vi "Calibration.vi"() -> ()   [LabVIEW 2016]
uses:
  controls/EnumFGVHDT.ctl
  controls/Enum.ctl
  Course Project/support/Message Queue/Message Cluster.ctl
  <vilib>/rvi/errors/niLvFpgaAdjustHostInterfaceError.vi
  <vilib>/Utility/config.llb/Read Key (Double).vi
  <vilib>/Utility/config.llb/Read Key (String).vi
  <vilib>/Utility/config.llb/Read Key (U32).vi
  <vilib>/Utility/config.llb/Write Key (Double).vi
  <vilib>/Utility/config.llb/Write Key (String).vi
  <vilib>/Utility/config.llb/Write Key (Boolean).vi
  controls/FPGAVIreferenceTypeDef.ctl
  <vilib>/rvi/interface/nirviReadWriteControl/nirviReadWriteControl.xnode
  FPGA Bitfiles/qnmController797_usbRio80MHz_1.lvbitx
  <vilib>/regexp/Match Regular Expression.xnode
  Course Project/support/Message Queue/Message Queue.lvlib
  Course Project/support/User Event - Stop/User Event - Stop.lvlib
  <vilib>/Utility/config.llb/NI_LVConfig.lvlib
  NiFpgaLv.dll
panel:
  in  "Actions":i32(listbox)
  in  "Menus":T1(tab)
  in  "ActionsCalib":T2={"Calibrations"=0, "Calib parameters"={"Sensitivity"={"Sens X"=1e-07, "Sens Y"=1e-07, "Sens Z"=2e-08}, "Range"={"Range X"=0.0, "Range Y"=0.0, "Range Z"=0.0}, "Gain"={"HV gain X"=0.0, "HV gain Y"=0.0, "HV gain Z"=0.0}}, "EditList"={"Add"=FALSE, "Copy"=FALSE, "Delete"=FALSE, "Up"=FALSE, "Down"=FALSE, "Apply"=FALSE}} {"Calib parameters"."Gain"."HV gain X" min=0.0 max=44.0 step=1.0 format="%#.0f"; "Calib parameters"."Gain"."HV gain Y" min=0.0 max=44.0 step=1.0 format="%#.0f"; "Calib parameters"."Gain"."HV gain Z" min=0.0 max=44.0 step=1.0 format="%#.0f"; "Calib parameters"."Range"."Range X" format="%#_3pm"; "Calib parameters"."Range"."Range Y" format="%#_3pm"; "Calib parameters"."Range"."Range Z" format="%#_3pm"; "Calib parameters"."Sensitivity"."Sens X" format="%#.2pm/V"; "Calib parameters"."Sensitivity"."Sens Y" format="%#.2pm/V"; "Calib parameters"."Sensitivity"."Sens Z" format="%#.2pm/V"}
  in  "OpenHysteresisVi":bool
  out "fwd":dbl[](array[numeric]) format="%#.4g"
  out "bwd":dbl[](array[numeric]) format="%#.4g"
  in  "Hyst Compens":cluster{"Hysteresis Comp":bool}={"Hysteresis Comp"=TRUE}
  in  "Voltage Limits":cluster{"X":dbl, "Y":dbl, "Z":dbl}={"X"=10.0, "Y"=10.0, "Z"=10.0} {"Z" min=-10.0 max=10.0 format="%#_3pV"; "Y" min=-10.0 max=10.0 format="%#_3pV"; "X" min=-10.0 max=10.0 format="%#_3pV"}
  in  "HV":T3
  in  "Analogs":T4={"AI"={"0"=TRUE, "1"=TRUE, "2"=TRUE, "3"=TRUE, "4"=TRUE, "5"=TRUE, "6"=TRUE}, "AO"={"0"=TRUE, "1"=TRUE, "2"=TRUE, "3"=TRUE, "4"=TRUE, "5"=TRUE, "6"=TRUE}}
  in  "ScannerConfig":T5={"Speed config"=FALSE, "Time Constant (us)"=40} {"Time Constant (us)" format="%#.0f"}
  # "Piezo Calibration"
  # "Polynom coeff : a+bx +cx2+dx3"
  # "Hysteresis Compensation"
  # "High Voltage"
  # "between -10V..+10V"
  # "AI/AO inversion"
  # "Non inverted"
  # "Inverted"
  # "Non inverted"
  # "Inverted"
  # "Scanner Configuration"
  # "- slow"
  # "- fast"
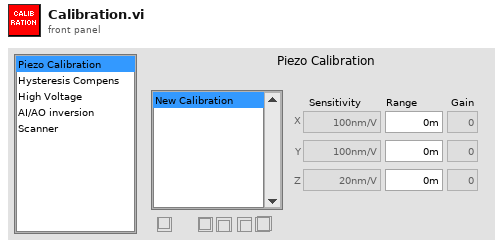
[diagram p1: front panel]
types:
  T1 = enum32{"Piezo Calibration", "Hyst Compens", "High Voltage", "Hyst Compens 2", "Hyst Compens 3", "High Voltage 2", "High Voltage 3", "High Voltage 4", "High Voltage 5"}
  T2 = cluster{"Calibrations":i32, "Calib parameters":cluster{"Sensitivity":cluster{"Sens X":dbl, "Sens Y":dbl, "Sens Z":dbl}, "Range":cluster{"Range X":dbl, "Range Y":dbl, "Range Z":dbl}, "Gain":cluster{"HV gain X":dbl, "HV gain Y":dbl, "HV gain Z":dbl}}, "EditList":cluster{"Add":bool, "Copy":bool, "Delete":bool, "Up":bool, "Down":bool, "Apply":bool}}
  T3 = cluster{"X":bool, "Y":bool, "Z":bool, "X 2":bool, "Y 2":bool, "Z 2":bool}
  T4 = cluster{"AI":cluster{"0":bool, "1":bool, "2":bool, "3":bool, "4":bool, "5":bool, "6":bool}, "AO":cluster{"0":bool, "1":bool, "2":bool, "3":bool, "4":bool, "5":bool, "6":bool}}
  T5 = cluster{"Speed config":bool, "Time Constant (us)":u16}
  T6 = typedef "EnumFGVHDT.ctl" = enum16{"Init", "Read", "Write", "Push", "Pop"}
  T7 = typedef "Message Queue.lvlib/All Message Queues.ctl" = cluster{"IU":refnum<queue>}
  T8 = typedef "Enum.ctl" = enum16{"Init", "Read", "Write"}
  T9 = enum16{"fractional", "engineering", "exponential"}
  T10 = typedef "Message Queue.lvlib/Message Cluster.ctl" = cluster{"Message":string, "Données de message":variant}
  T11 = cluster{"Sensitivity":cluster{"Sens Z":dbl, "Sens Y":dbl, "Sens X":dbl}, "Range":cluster{"Range Z":dbl, "Range Y":dbl, "Range X":dbl}, "HV gain":cluster{"HV gain Z":i32, "HV gain Y":i32, "HV gain X":i32}}
  T12 = cluster{"calibName":string[], "calibParameters":cluster{"Sensitivity":cluster{"Sens X":dbl, "Sens Y":dbl, "Sens Z":dbl}, "Range":cluster{"Range X":dbl, "Range Y":dbl, "Range Z":dbl}, "HV gain":cluster{"HV gain X":dbl, "HV gain Y":dbl, "HV gain Z":dbl}}[], "calibIndex":i32}
  T13 = typedef "NI_LVConfig.lvlib/Config Data RefNum.ctl" = refnum<k1>
  T14 = cluster{"Sensitivity":cluster{"Sens X":dbl, "Sens Y":dbl, "Sens Z":dbl}, "Range":cluster{"Range X":dbl, "Range Y":dbl, "Range Z":dbl}, "HV gain":cluster{"HV gain X":dbl, "HV gain Y":dbl, "HV gain Z":dbl}}[]
  T15 = cluster{"Sensitivity":cluster{"Sens X":dbl, "Sens Y":dbl, "Sens Z":dbl}, "Range":cluster{"Range X":dbl, "Range Y":dbl, "Range Z":dbl}, "HV gain":cluster{"HV gain X":dbl, "HV gain Y":dbl, "HV gain Z":dbl}}
  T16 = cluster{"Sens X":dbl, "Sens Y":dbl, "Sens Z":dbl}
  T17 = cluster{"Range X":dbl, "Range Y":dbl, "Range Z":dbl}
  T18 = cluster{"HV gain X":dbl, "HV gain Y":dbl, "HV gain Z":dbl}
  T19 = cluster{"Sensitivity":cluster{"Sens X":dbl, "Sens Y":dbl, "Sens Z":dbl}, "Range":cluster{"Range X":dbl, "Range Y":dbl, "Range Z":dbl}, "Gain":cluster{"HV gain X":dbl, "HV gain Y":dbl, "HV gain Z":dbl}}
  T20 = typedef "FPGAVIreferenceTypeDef.ctl" = refnum<k20>
  T21 = cluster{"0":bool, "1":bool, "2":bool, "3":bool, "4":bool, "5":bool, "6":bool}
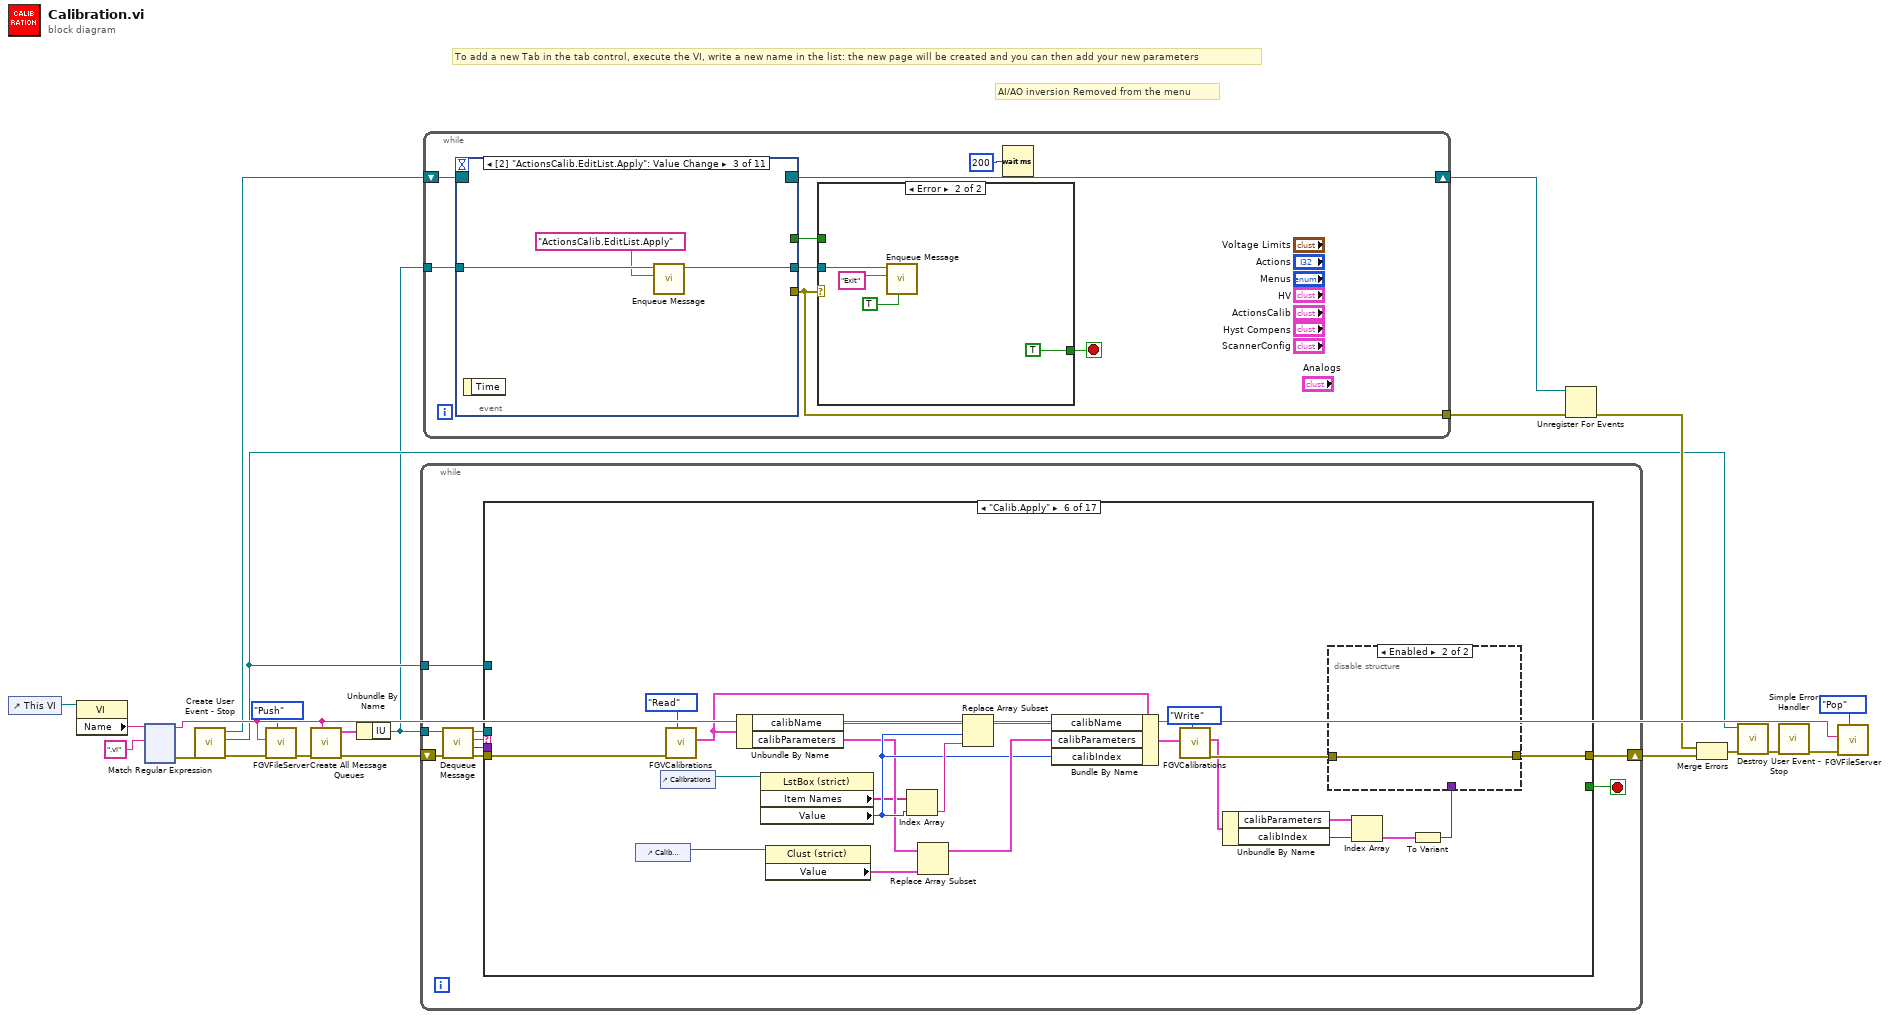
[diagram p0: block diagram]
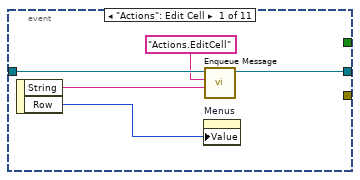
[diagram p3: hidden frame]
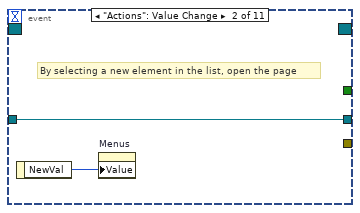
[diagram p4: hidden frame]
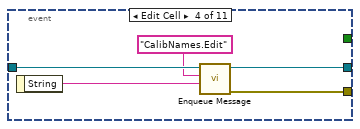
[diagram p5: hidden frame]
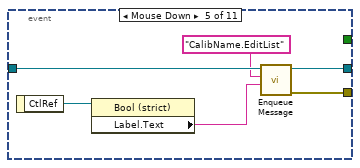
[diagram p6: hidden frame]
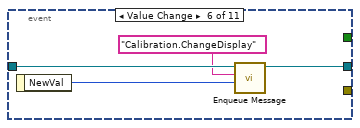
[diagram p7: hidden frame]
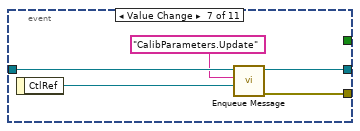
[diagram p8: hidden frame]
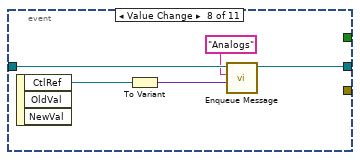
[diagram p9: hidden frame]
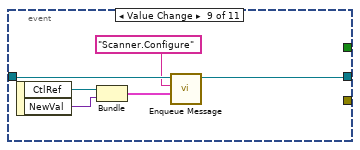
[diagram p10: hidden frame]
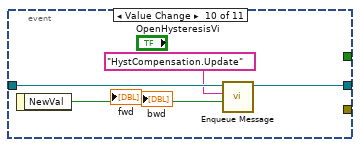
[diagram p11: hidden frame]
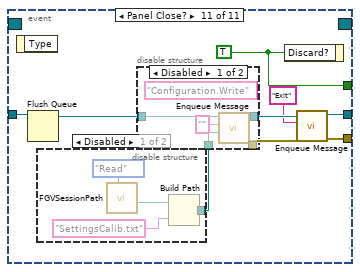
[diagram p12: hidden frame]
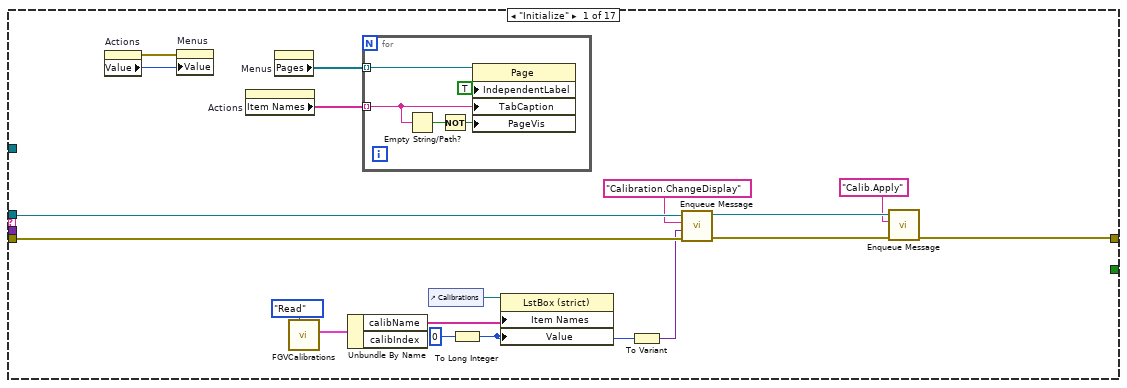
[diagram p15: hidden frame]
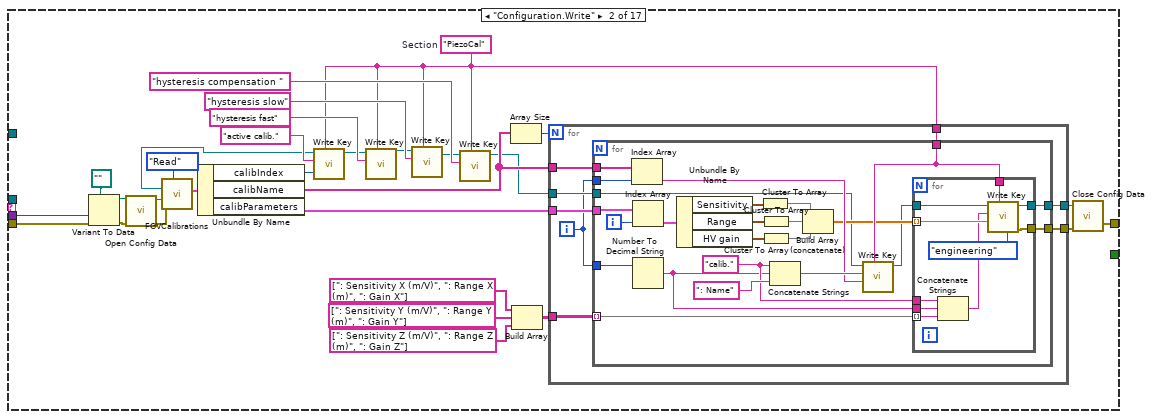
[diagram p16: hidden frame]
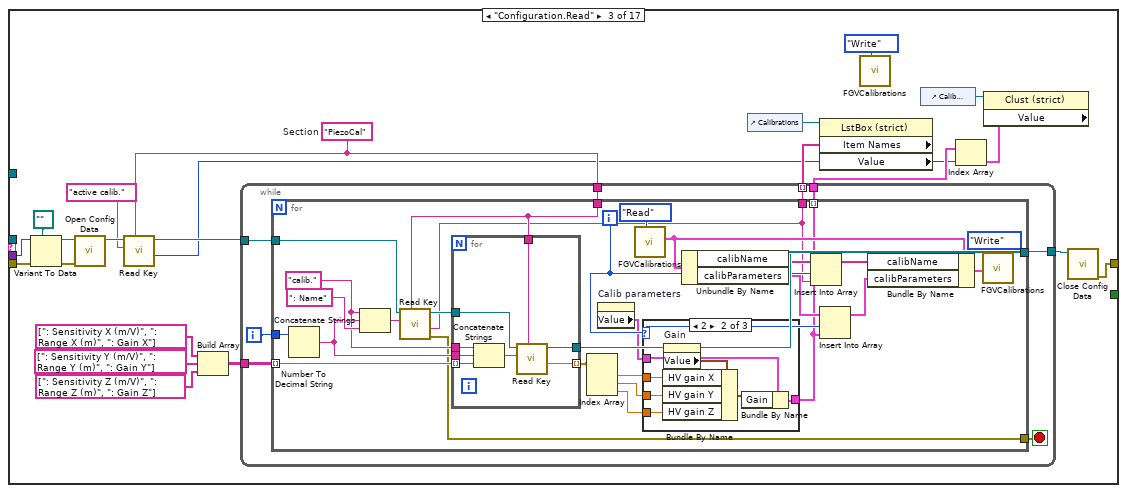
[diagram p17: hidden frame]
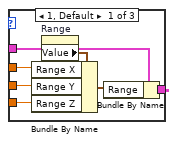
[diagram p18: hidden frame]
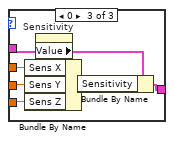
[diagram p19: hidden frame]
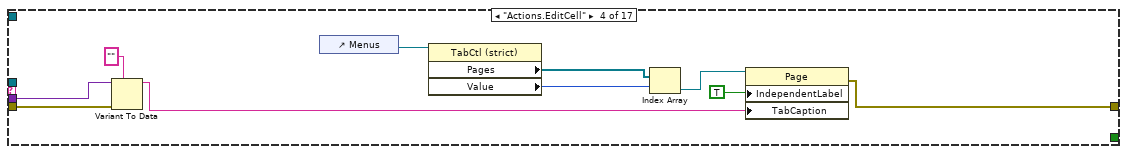
[diagram p20: hidden frame]
diagram:
  # "AI/AO inversion Removed from the menu"
  # "To add a new Tab in the tab control, execute the VI, write a new name in the list: the new page will be created and you can then add your new parameters"
  n1 = control-ref of="This VI"() -> (w9:refnum<vi>)
  n2 = property class="VI"(reference=w9) -> ("Name"=w8:string)  [unwired: 1 in, 2 out]
  n3 = xnode "Match Regular Expression"("input string"=w8, "regular expression"=".vi") -> ("before match"=w21:string, "error out"=w6:errorcluster)  [unwired: 4 in, 3 out]
  n4 = call "Create User Event - Stop.vi"("entrée d'erreur (pas d'erreur)"=w6) -> ("sortie d'erreur"=w4:errorcluster, "Événement utilisateur - Arrêt"=w17:refnum<user-event>, "Refnum Enregistrement à l'événement Arrêt"=w14:refnum<event-registration>)  [unwired: 8 in]
  n5 = call "FGVFileServer.vi"("Enum"=EnumFGVHDT."Push", "error in"=w4, "New VI"=w21) -> ("error out"=w3:errorcluster)  [unwired: 7 in, 1 out]
  n6 = call "Create All Message Queues.vi"("QueueName"=w21, "ErrorIn"=w3) -> ("ErrorOut"=w10:errorcluster, "MessageQueueOut"=w11:T7)  [unwired: 8 in]
  n7 = Unbundle By Name(w11) -> ("IU"=w13:refnum<queue>)
  n8 = while {
    tunnel: w13 -> [w22]
    tunnel: w17 -> [w28]
    shift-right: [w29] -> w12
    shift-left: w10 -> [w27]
    stop <- w30 stop-if-true
    n9 = call "Dequeue Message.vi"("entrée d'erreur (pas d'erreur)"=w27, "File d'attente de messages"=w22) -> ("sortie d'erreur"=w26:errorcluster, "Données de message"=w24:variant, "Message"=w25:string, "File d'attente de message dup."=w23:refnum<queue>)  [unwired: 6 in]
    n10 = case "Conditions des messages" shown="\"Calib.Apply\"" w25 {
      selector: w25 -> [_ _ _ _ _ _ _ _ _ _ _ _ _ _ _ _ w601]
      tunnel: w23 -> [w47 _ _ _ w242 _ _ _ _ w403 _ _ _ w558 _ w597 _]
      tunnel: w26 -> [w41 w62 w148 w222 w233 w258 w296 w302 w393 w398 w414 w517 w525 w557 w590 w593 _]
      tunnel: [w38 w59 w128 w217 w235 w256 w290 w298 w386 w399 w411 w517 w519 w542 w585 w594 w599] -> w29
      tunnel: [_ _ _ _ _ _ _ _ _ _ _ _ _ _ _ TRUE _] -> w30
      tunnel: w24 -> [_ w55 w147 w221 _ _ w295 w301 w392 w395 w413 _ w526 w556 w589 _ _]
      tunnel: w28 -> [_ _ _ _ _ _ _ _ _ _ _ _ _ _ _ w592 _]
      frame "Initialize" {
        n11 = property on="Actions" class="LstBox (strict)"() -> (error out=w43:errorcluster, "Value"=w44:i32)  [unwired: 2 in, 1 out]
        n12 = property on="Menus" class="TabCtl (strict)"(error in=w43, "Value"=w44) -> ()  [unwired: 1 in, 2 out]
        n13 = property on="Actions" class="LstBox (strict)"() -> ("Item Names"=w46:string[])  [unwired: 2 in, 2 out]
        n14 = property on="Menus" class="TabCtl (strict)"() -> ("Pages"=w45:refnum<vi>[])  [unwired: 2 in, 2 out]
        n15 = call "FGVCalibrations.vi"("Enum"=Enum."Read") -> ("calibOut"=w34:T12)  [unwired: 9 in, 1 out]
        n16 = Unbundle By Name(w34) -> ("calibName"=w32:string[])  [unwired: 1 out]
        n17 = for {
          tunnel: w45 -> [w53] mode=indexing
          tunnel: w46 -> [w49] mode=indexing
          n18 = Empty String/Path?(string/path=w49) -> (empty?=w51:bool)
          n19 = Not(x=w51) -> (.not. x?=w50:bool)
          n20 = property class="Page"(reference=w53, "IndependentLabel"=TRUE ("Étiquette indépendante"), "TabCaption"=w49, "PageVis"=w50) -> ()  [unwired: 1 in, 2 out]
        }
        n21 = control-ref of="Calibrations"() -> (w33:refnum<vi>)
        n22 = To Long Integer(number=0) -> (32bit integer=w40:i32)
        n23 = property class="LstBox (strict)"(reference=w33, "Item Names"=w32, "Value"=w40) -> ()  [unwired: 1 in, 2 out]
        n24 = To Variant(anything=w40) -> (Variant=w36:variant)
        n25 = call "Enqueue Message.vi"("error in"=w41, "Data"=w36, "Message"="Calibration.ChangeDisplay", "Queue"=w47) -> ("error out"=w39:errorcluster, "Queue dup."=w48:refnum<queue>)  [unwired: 6 in]
        n26 = call "Enqueue Message.vi"("error in"=w39, "Message"="Calib.Apply", "Queue"=w48) -> ("error out"=w38:errorcluster)  [unwired: 7 in, 1 out]
      }
      frame "Configuration.Write" {
        w66 = "PiezoCal"  # Section
        n27 = Variant To Data(error in=w62, type=path "" ("appended path"), Variant=w55) -> (data=w56:path, error out=w61:errorcluster)
        n28 = call <vilib>:"Open Config Data.vi"("error in (no error)"=w61, "configuration file path"=w56) -> ("error out"=w58:errorcluster, "refnum"=w57:T13)  [unwired: 1 in, 7 out]
        n29 = call "FGVCalibrations.vi"("Enum"=Enum."Read", "error in"=w58) -> ("calibOut"=w74:T12)  [unwired: 8 in, 1 out]
        n30 = Unbundle By Name(w74) -> ("calibIndex"=w64:i32, "calibName"=w78:string[], "calibParameters"=w65:T14)
        n31 = call-poly <vilib>:"Write Key.vi"("section"=w66, "value"=w64, "key"="active calib.", "refnum"=w57) -> ("refnum out"=w67:T13)  [unwired: 4 in, 3 out]
        n32 = call-poly <vilib>:"Write Key.vi"("section"=w66, "key"="hysteresis fast", "refnum"=w67) -> ("refnum out"=w68:T13)  [unwired: 2 in, 6 out]
        n33 = call-poly <vilib>:"Write Key.vi"("section"=w66, "key"="hysteresis slow", "refnum"=w68) -> ("refnum out"=w69:T13)  [unwired: 2 in, 6 out]
        n34 = call-poly <vilib>:"Write Key.vi"("section"=w66, "key"="hysteresis compensation ", "refnum"=w69) -> ("refnum out"=w76:T13)  [unwired: 2 in, 6 out]
        n35 = Array Size(array=w78) -> (size(s)=w77:i32)
        n36 = Build Array(string[] [": Sensitivity X (m/V)", ": Range X (m)", ": Gain X"] ("Array"), string[] [": Sensitivity Y (m/V)", ": Range Y (m)", ": Gain Y"] ("Array"), string[] [": Sensitivity Z (m/V)", ": Range Z (m)", ": Gain Z"] ("Array")) -> (w79:string[][])
        n37 = for {
          N: w77 -> [_]
          tunnel: w65 -> [w90]
          tunnel: w79 -> [w89]
          tunnel: w66 -> [w88]
          tunnel: w78 -> [w86]
          tunnel: w76 -> [w87]
          tunnel: [w84] -> w60
          tunnel: [w83] -> w54
          i -> [w85]
          n38 = for {
            tunnel: w86 -> [w114]
            tunnel: w90 -> [w110]
            tunnel: w88 -> [w108]
            tunnel: w89 -> [w93] mode=indexing
            tunnel: w87 -> [w100]
            tunnel: w85 -> [w98]
            tunnel: w85 -> [w97]
            tunnel: [w92] -> w84
            tunnel: [w91] -> w83
            i -> [w96]
            w95 = "calib."
            n39 = Index Array(array=w114, index=w97) -> (element=w111:string)
            n40 = Index Array(array=w110, index=w96) -> (element=w109:T15)
            n41 = Number To Decimal String(number=w98) -> (decimal integer string=w94:string)  [unwired: 1 in]
            n42 = Unbundle By Name(w109) -> ("Sensitivity"=w107:T16, "Range"=w105:T17, "HV gain"=w106:T18)
            n43 = Cluster To Array(cluster=w107) -> (array=w104:dbl[])
            n44 = Cluster To Array(cluster=w105) -> (array=w103:dbl[])
            n45 = Cluster To Array(cluster=w106) -> (array=w102:dbl[])
            n46 = Concatenate Strings(w95, w94, ": Name") -> (w112:string)
            n47 = Build Array (concatenate)(w104, w103, w102) -> (w101:dbl[])
            n48 = call-poly <vilib>:"Write Key.vi"("section"=w108, "value"=w111, "key"=w112, "refnum"=w100) -> ("refnum out"=w99:T13)  [unwired: 2 in, 5 out]
            n49 = for {
              tunnel: w108 -> [w124]
              tunnel: w101 -> [w123] mode=indexing
              tunnel: w99 -> [w122]
              tunnel: w95 -> [w121]
              tunnel: w94 -> [w120]
              tunnel: w93 -> [w119] mode=indexing
              tunnel: [w117] -> w92
              tunnel: [w116] -> w91
              n50 = Concatenate Strings(w121, w120, w119) -> (w118:string)
              n51 = call-poly <vilib>:"Write Key.vi"("format (fractional)"=T9."engineering", "section"=w124, "value"=w123, "key"=w118, "refnum"=w122) -> ("error out"=w117:errorcluster, "refnum out"=w116:T13)  [unwired: 3 in, 2 out]
            }
          }
        }
        n52 = call <vilib>:"Close Config Data.vi"("error in (no error)"=w60, "refnum"=w54) -> ("error out"=w59:errorcluster)  [unwired: 1 in, 8 out]
      }
      frame "Configuration.Read" {
        w141 = "PiezoCal"  # Section
        n53 = Variant To Data(error in=w148, type=path "" ("appended path"), Variant=w147) -> (data=w149:path, error out=w150:errorcluster)
        n54 = call <vilib>:"Open Config Data.vi"("error in (no error)"=w150, "configuration file path"=w149) -> ("refnum"=w152:T13)  [unwired: 1 in, 8 out]
        n55 = call-poly <vilib>:"Read Key.vi"("section"=w141, "key"="active calib.", "refnum"=w152) -> ("value"=w126:u32, "refnum out"=w131:T13)  [unwired: 5 in, 2 out]
        n56 = Build Array(string[] [": Sensitivity X (m/V)", ": Range X (m)", ": Gain X"] ("Array"), string[] [": Sensitivity Y (m/V)", ": Range Y (m)", ": Gain Y"] ("Array"), string[] [": Sensitivity Z (m/V)", ": Range Z (m)", ": Gain Z"] ("Array")) -> (w143:string[][])
        n57 = while {
          tunnel: w143 -> [w160]
          tunnel: w141 -> [w159]
          tunnel: w131 -> [w158]
          tunnel: [w156] -> w140
          tunnel: [w155] -> w130 mode=indexing
          tunnel: [w153] -> w127
          i -> [w157]
          stop <- w154 stop-if-true
          n58 = for {
            tunnel: w159 -> [w185]
            tunnel: w160 -> [w179] mode=indexing
            tunnel: w158 -> [w184]
            tunnel: w157 -> [w182]
            tunnel: [w178] -> w156
            tunnel: [w163] -> w155
            tunnel: [w162] -> w154
            tunnel: [w161] -> w153 mode=indexing
            i -> [w170]
            w181 = "calib."
            n59 = Number To Decimal String(number=w182) -> (decimal integer string=w180:string)  [unwired: 1 in]
            n60 = Concatenate Strings(w181, w180, ": Name") -> (w186:string)
            n61 = call-poly <vilib>:"Read Key.vi"("section"=w185, "key"=w186, "refnum"=w184) -> ("error out"=w162:errorcluster, "value"=w163:string, "refnum out"=w183:T13)  [unwired: 5 in, 1 out]
            n62 = for {
              tunnel: w185 -> [w216]
              tunnel: w183 -> [w215]
              tunnel: w181 -> [w214]
              tunnel: w180 -> [w213]
              tunnel: w179 -> [w212] mode=indexing
              tunnel: [w210] -> w178
              tunnel: [w209] -> w177 mode=indexing
              n63 = Concatenate Strings(w214, w213, w212) -> (w211:string)
              n64 = call-poly <vilib>:"Read Key.vi"("section"=w216, "key"=w211, "refnum"=w215) -> ("value"=w209:dbl, "refnum out"=w210:T13)  [unwired: 5 in, 2 out]
            }
            n65 = Index Array(array=w177) -> (element #1=w167:dbl, element #2=w166:dbl, element #3=w165:dbl)  [unwired: 3 in]
            n66 = property on="Calib parameters" class="Clust (strict)"() -> ("Value"=w169:T19)  [unwired: 2 in, 2 out]
            n67 = call "FGVCalibrations.vi"("Enum"=Enum."Read") -> ("calibOut"=w173:T12)  [unwired: 9 in, 1 out]
            n68 = case shown="2" w170 {
              tunnel: [w192 w199 w206] -> w161
              tunnel: w169 -> [w191 w198 w205]
              tunnel: w167 -> [w190 w197 w204]
              tunnel: w166 -> [w189 w196 w203]
              tunnel: w165 -> [w188 w195 w202]
              frame 1, Default {
                n69 = property on="Range" class="Clust (strict)"() -> ("Value"=w194:T17)  [unwired: 2 in, 2 out]
                n70 = Bundle By Name(cluster=w194, "Range X"=w190, "Range Y"=w189, "Range Z"=w188) -> (w193:T17)
                n71 = Bundle By Name(cluster=w191, "Range"=w193) -> (w192:T19)
              }
              frame 2 {
                n72 = property on="Gain" class="Clust (strict)"() -> ("Value"=w201:T18)  [unwired: 2 in, 2 out]
                n73 = Bundle By Name(cluster=w201, "HV gain X"=w197, "HV gain Y"=w196, "HV gain Z"=w195) -> (w200:T18)
                n74 = Bundle By Name(cluster=w198, "Gain"=w200) -> (w199:T19)
              }
              frame 0 {
                n75 = property on="Sensitivity" class="Clust (strict)"() -> ("Value"=w208:T16)  [unwired: 2 in, 2 out]
                n76 = Bundle By Name(cluster=w208, "Sens X"=w204, "Sens Y"=w203, "Sens Z"=w202) -> (w207:T16)
                n77 = Bundle By Name(cluster=w205, "Sensitivity"=w207) -> (w206:T19)
              }
            }
            n78 = Unbundle By Name(w173) -> ("calibName"=w164:string[], "calibParameters"=w171:T14)
            n79 = Insert Into Array(array=w164, index=w170, new element=w163) -> (w172:string[])
            n80 = Insert Into Array(array=w171, index=w170, new element=w161) -> (w168:T14)
            n81 = Bundle By Name(cluster=w173, "calibName"=w172, "calibParameters"=w168) -> (w174:T12)
            n82 = call "FGVCalibrations.vi"("Enum"=Enum."Write", "calibIn"=w174) -> ()  [unwired: 8 in, 2 out]
          }
        }
        n83 = control-ref of="Calibrations"() -> (w136:refnum<vi>)
        n84 = control-ref of="Calibrations"() -> (w137:refnum<vi>)
        n85 = control-ref of="Calibrations"() -> (w138:refnum<vi>)
        n86 = control-ref of="Calibrations"() -> (w139:refnum<vi>)
        n87 = property class="LstBox (strict)"(reference=w136, "Item Names"=w130, "Value"=w126) -> ()  [unwired: 1 in, 2 out]
        n88 = property class="LstBox (strict)" props=["Item Names", "Value"](reference=w137) -> ()  [unwired: 1 in, 4 out]
        n89 = property class="LstBox (strict)" props=["Item Names", "Value"](reference=w138) -> ()  [unwired: 1 in, 4 out]
        n90 = property class="LstBox (strict)" props=["Item Names", "Value"](reference=w139) -> ()  [unwired: 1 in, 4 out]
        n91 = call "FGVCalibrations.vi"("Enum"=Enum."Write") -> ()  [unwired: 9 in, 2 out]
        n92 = control-ref of="Calib parameters"() -> (w132:refnum<vi>)
        n93 = control-ref of="Calib parameters"() -> (w133:refnum<vi>)
        n94 = control-ref of="Calib parameters"() -> (w134:refnum<vi>)
        n95 = control-ref of="Calib parameters"() -> (w135:refnum<vi>)
        n96 = Index Array(array=w127, index=w126) -> (element=w125:T19)
        n97 = property class="Clust (strict)"(reference=w132, "Value"=w125) -> ()  [unwired: 1 in, 2 out]
        n98 = property class="Clust (strict)" props=["Value"](reference=w133) -> ()  [unwired: 1 in, 3 out]
        n99 = property class="Clust (strict)" props=["Value"](reference=w134) -> ()  [unwired: 1 in, 3 out]
        n100 = property class="Clust (strict)" props=["Value"](reference=w135) -> ()  [unwired: 1 in, 3 out]
        n101 = call <vilib>:"Close Config Data.vi"("refnum"=w140) -> ("error out"=w128:errorcluster)  [unwired: 2 in, 8 out]
      }
      frame "Actions.EditCell" {
        n102 = Variant To Data(error in=w222, type="" ("String"), Variant=w221) -> (data=w219:string)  [unwired: 1 out]
        n103 = control-ref of="Menus"() -> (w224:refnum<vi>)
        n104 = property class="TabCtl (strict)"(reference=w224) -> ("Pages"=w225:refnum<vi>[], "Value"=w218:T1)  [unwired: 1 in, 2 out]
        n105 = Index Array(array=w225, index=w218) -> (element=w226:refnum<vi>)
        n106 = property class="Page"(reference=w226, "IndependentLabel"=TRUE ("Étiquette indépendante"), "TabCaption"=w219) -> (error out=w217:errorcluster)  [unwired: 1 in, 1 out]
      }
      frame "ActionsCalib.EditList.Apply" {
        n107 = call "Enqueue Message.vi"("error in"=w233, "Message"="Calib.Apply", "Queue"=w242) -> ("error out"=w232:errorcluster)  [unwired: 7 in, 1 out]
        n108 = control-ref of="Calibrations"() -> (w237:refnum<vi>)
        n109 = property class="LstBox (strict)"(reference=w237, error in=w232) -> (reference out=w236:refnum<vi>, "Number of Rows"=w240:u32, "Value"=w228:i32)  [unwired: 1 out]
        n110 = call "FGVCalibrations.vi"("Enum"=Enum."Read") -> ("calibOut"=w229:T12)  [unwired: 9 in, 1 out]
        n111 = Bundle By Name(cluster=w229, "calibIndex"=w228) -> (w227:T12)
        n112 = Initialize Array(0 ("cas faux"), w240) -> (w241:i32[])
        n113 = for {
          N: w240 -> [_]
          tunnel: w228 -> [w243]
          shift-right: [w245] -> w238
          shift-left: w241 -> [w250]
          i -> [w244]
          n114 = Equal?(x=w244, y=w243) -> (x = y?=w249:bool)
          n115 = Select(t=1 ("nouvel élément/sous-tableau"), s=w249, f=0 ("cas faux")) -> (s? t:f=w246:i32)
          n116 = Replace Array Subset(array=w250, new element=w246, index=w244) -> (w245:i32[])
        }
        n117 = call "FGVCalibrations.vi"("Enum"=Enum."Write", "calibIn"=w227) -> ()  [unwired: 8 in, 2 out]
        n118 = property class="LstBox (strict)"(reference=w236, "Item Symbols"=w238) -> (error out=w235:errorcluster)  [unwired: 1 in, 1 out]
      }
      frame "Calib.Apply" {
        n119 = control-ref of="Calib parameters"() -> (w263:refnum<vi>)
        n120 = control-ref of="Calibrations"() -> (w262:refnum<vi>)
        n121 = call "FGVCalibrations.vi"("Enum"=Enum."Read", "error in"=w258) -> ("calibOut"=w270:T12)  [unwired: 8 in, 1 out]
        n122 = Unbundle By Name(w270) -> ("calibName"=w259:string[], "calibParameters"=w265:T14)
        n123 = property class="LstBox (strict)"(reference=w262) -> ("Item Names"=w261:string[], "Value"=w266:i32)  [unwired: 1 in, 2 out]
        n124 = property class="Clust (strict)"(reference=w263) -> ("Value"=w264:T19)  [unwired: 1 in, 2 out]
        n125 = Index Array(array=w261, index=w266) -> (element=w268:string)
        n126 = Replace Array Subset(array=w265, new element=w264) -> (w267:T14)  [unwired: 1 in]
        n127 = Replace Array Subset(array=w259, new element=w268, index=w266) -> (w260:string[])
        n128 = Bundle By Name(cluster=w270, "calibName"=w260, "calibParameters"=w267, "calibIndex"=w266) -> (w269:T12)
        n129 = call "FGVCalibrations.vi"("Enum"=Enum."Write", "calibIn"=w269) -> ("error out"=w257:errorcluster, "calibOut"=w255:T12)  [unwired: 8 in]
        n130 = Unbundle By Name(w255) -> ("calibParameters"=w254:T14, "calibIndex"=w253:i32)
        n131 = Index Array(array=w254, index=w253) -> (element=w252:T15)
        n132 = To Variant(anything=w252) -> (Variant=w251:variant)
        n133 = disable-structure shown="Enabled" {
          disable-tunnel: w257 -> [w275 w281]
          disable-tunnel: [w274 w281] -> w256
          disable-tunnel: w251 -> [w273 _]
          frame Disabled {
            n134 = Obtain Queue(name (unnamed)="Scan", element data type=T10 {"Message"="", "Données de message"=variant} ("Cluster Message"), error in (no error)=w275) -> (queue out=w280:refnum<queue>, error out=w277:errorcluster)  [unwired: 2 in, 1 out]
            n135 = call "Enqueue Message.vi"("error in"=w277, "Data"=w273, "Message"="Calibration.Update", "Queue"=w280) -> ("error out"=w274:errorcluster)  [unwired: 6 in, 1 out]
          }
          frame Enabled {
          }
        }
      }
      frame "CalibNames.Edit" {
        n136 = Variant To Data(error in=w296, type="", Variant=w295) -> (data=w284:string, error out=w294:errorcluster)
        n137 = call "FGVCalibrations.vi"("Enum"=Enum."Read", "error in"=w294) -> ("error out"=w291:errorcluster, "calibOut"=w288:T12)  [unwired: 8 in]
        n138 = control-ref of="Calibrations"() -> (w287:refnum<vi>)
        n139 = property class="LstBox (strict)"(reference=w287) -> ("Value"=w285:i32)  [unwired: 1 in, 2 out]
        n140 = Unbundle By Name(w288) -> ("calibName"=w286:string[])
        n141 = Replace Array Subset(array=w286, new element=w284, index=w285) -> (w283:string[])
        n142 = Bundle By Name(cluster=w288, "calibName"=w283) -> (w289:T12)
        n143 = call "FGVCalibrations.vi"("Enum"=Enum."Write", "error in"=w291, "calibIn"=w289) -> ("error out"=w290:errorcluster)  [unwired: 7 in, 1 out]
      }
      frame "CalibName.EditList" {
        n144 = Variant To Data(error in=w302, type="", Variant=w301) -> (data=w299:string, error out=w297:errorcluster)
        n145 = case shown="\"Down\", \"Up\"" w299 {
          selector: w299 -> [_ _ _ w380]
          tunnel: [w304 w332 w341 w358] -> w298
          tunnel: w297 -> [w303 w331 w349 w357]
          frame "Copy", Default {
            n146 = call "FGVCalibrations.vi"("Enum"=Enum."Read", "error in"=w303) -> ("calibOut"=w310:T12)  [unwired: 8 in, 1 out]
            n147 = control-ref of="Calibrations"() -> (w319:refnum<vi>)
            n148 = Unbundle By Name(w310) -> ("calibParameters"=w309:T14)
            n149 = property class="LstBox (strict)"(reference=w319) -> (reference out=w317:refnum<vi>, "Item Names"=w315:string[], "Value"=w308:i32)  [unwired: 1 in, 1 out]
            n150 = Index Array(array=w315, index=w308) -> (element=w316:string)
            n151 = Index Array(array=w309, index=w308) -> (element=w306:T15)
            n152 = Array Size(array=w315) -> (size(s)=w318:i32)
            n153 = Decrement(x=w318) -> (x-1=w307:i32)
            n154 = Insert Into Array(array=w315, index=w307, new element=w316) -> (w311:string[])
            n155 = Insert Into Array(array=w309, index=w307, new element=w306) -> (w305:T14)
            n156 = property class="LstBox (strict)"(reference=w317, "Item Names"=w311) -> ()  [unwired: 1 in, 2 out]
            n157 = Bundle By Name(cluster=w310, "calibName"=w311, "calibParameters"=w305) -> (w312:T12)
            n158 = call "FGVCalibrations.vi"("Enum"=Enum."Write", "calibIn"=w312) -> ("error out"=w304:errorcluster)  [unwired: 8 in, 1 out]
          }
          frame "Add" {
            w325 = "New Calibration" ("new element/subarray")
            # "Add Copy Delete Up Down Apply"
            n159 = control-ref of="Calibrations"() -> (w336:refnum<vi>)
            n160 = property class="LstBox (strict)"(reference=w336, error in=w331) -> (reference out=w335:refnum<vi>, "Item Names"=w333:string[])  [unwired: 1 out]
            n161 = call "FGVCalibrations.vi"("Enum"=Enum."Read") -> ("calibOut"=w327:T12)  [unwired: 9 in, 1 out]
            n162 = Unbundle By Name(w327) -> ("calibName"=w326:string[], "calibParameters"=w323:T14)
            n163 = Array Size(array=w333) -> (size(s)=w322:i32)
            n164 = Insert Into Array(array=w333, index=w322, new element=w325) -> (w334:string[])
            n165 = property class="LstBox (strict)"(reference=w335, "Item Names"=w334) -> (error out=w332:errorcluster)  [unwired: 1 in, 1 out]
            n166 = Insert Into Array(array=w323, index=w322, new element=T11 {"Sensitivity"={"Sens Z"=1e-07, "Sens Y"=1e-07, "Sens X"=1e-08}, "Range"={"Range Z"=4.4e-05, "Range Y"=4.4e-05, "Range X"=4.4e-06}, "HV gain"={"HV gain Z"=44, "HV gain Y"=44, "HV gain X"=44}} ("Calib parameters")) -> (w320:T14)
            n167 = Insert Into Array(array=w326, index=w322, new element=w325) -> (w324:string[])
            n168 = Bundle By Name(cluster=w327, "calibName"=w324, "calibParameters"=w320) -> (w328:T12)
            n169 = call "FGVCalibrations.vi"("Enum"=Enum."Write", "calibIn"=w328) -> ()  [unwired: 8 in, 2 out]
          }
          frame "Delete" {
            n170 = call "FGVCalibrations.vi"("Enum"=Enum."Read", "error in"=w349) -> ("calibOut"=w346:T12)  [unwired: 8 in, 1 out]
            n171 = Unbundle By Name(w346) -> ("calibName"=w344:string[], "calibParameters"=w345:T14)
            n172 = control-ref of="Calibrations"() -> (w354:refnum<vi>)
            n173 = property class="LstBox (strict)"(reference=w354) -> (reference out=w353:refnum<vi>, "Item Names"=w351:string[], "Value"=w338:i32)  [unwired: 1 in, 1 out]
            n174 = Delete From Array(array=w351, length=1, index=w338) -> (array with subset deleted=w352:string[])  [unwired: 1 out]
            n175 = Delete From Array(array=w345, length=1, index=w338) -> (array with subset deleted=w342:T14)  [unwired: 1 out]
            n176 = Delete From Array(array=w344, length=1, index=w338) -> (array with subset deleted=w343:string[])  [unwired: 1 out]
            n177 = property class="LstBox (strict)"(reference=w353, "Item Names"=w352) -> ()  [unwired: 1 in, 2 out]
            n178 = Bundle By Name(cluster=w346, "calibName"=w343, "calibParameters"=w342) -> (w347:T12)
            n179 = call "FGVCalibrations.vi"("Enum"=Enum."Write", "calibIn"=w347) -> ("error out"=w341:errorcluster)  [unwired: 8 in, 1 out]
          }
          frame "Down", "Up" {
            n180 = Equal?(x=w380, y="Up") -> (x = y?=w379:bool)
            n181 = control-ref of="Calibrations"() -> (w382:refnum<vi>)
            n182 = call "FGVCalibrations.vi"("Enum"=Enum."Read", "error in"=w357) -> ("calibOut"=w361:T12)  [unwired: 8 in, 1 out]
            n183 = property class="LstBox (strict)"(reference=w382) -> (reference out=w356:refnum<vi>, "Value"=w364:i32, "Item Names"=w376:string[])  [unwired: 1 in, 1 out]
            n184 = Unbundle By Name(w361) -> ("calibName"=w367:string[], "calibParameters"=w368:T14)
            n185 = Select(t=-1, s=w379, f=1) -> (s? t:f=w375:i32)
            n186 = Add(x=w364, y=w375) -> (x+y=w363:i32)
            n187 = Delete From Array(array=w376, index=w364) -> (deleted portion=w374:string, array with subset deleted=w355:string[])  [unwired: 1 in]
            n188 = Delete From Array(array=w367, index=w364) -> (deleted portion=w370:string, array with subset deleted=w366:string[])  [unwired: 1 in]
            n189 = Delete From Array(array=w368, index=w364) -> (deleted portion=w369:T15, array with subset deleted=w365:T14)  [unwired: 1 in]
            n190 = Insert Into Array(array=w355, index=w363, new element=w374) -> (w373:string[])
            n191 = Insert Into Array(array=w366, index=w363, new element=w370) -> (w360:string[])
            n192 = Insert Into Array(array=w365, index=w363, new element=w369) -> (w359:T14)
            n193 = property class="LstBox (strict)"(reference=w356, "Value"=w363, "Item Names"=w373) -> ()  [unwired: 1 in, 2 out]
            n194 = Bundle By Name(cluster=w361, "calibName"=w360, "calibParameters"=w359) -> (w362:T12)
            n195 = call "FGVCalibrations.vi"("Enum"=Enum."Write", "calibIn"=w362) -> ("error out"=w358:errorcluster)  [unwired: 8 in, 1 out]
          }
        }
      }
      frame "Calibration.ChangeDisplay" {
        # "replace or insert"
        n196 = Variant To Data(error in=w393, type=0, Variant=w392) -> (data=w384:i32, error out=w391:errorcluster)
        n197 = call "FGVCalibrations.vi"("Enum"=Enum."Read", "error in"=w391) -> ("calibOut"=w385:T12)  [unwired: 8 in, 1 out]
        n198 = Unbundle By Name(w385) -> ("calibParameters"=w387:T14)  [unwired: 1 out]
        n199 = Index Array(array=w387, index=w384) -> (element=w388:T15)
        n200 = control-ref of="Calib parameters"() -> (w389:refnum<vi>)
        n201 = property class="Clust (strict)"(reference=w389, "Value"=w388) -> (error out=w386:errorcluster)  [unwired: 1 in, 1 out]
      }
      frame "CalibParameters.Update" {
        n202 = Variant To Data(error in=w398, type=refnum<vi> refnum ("CtlRef"), Variant=w395) -> (data=w394:refnum<vi>, error out=w397:errorcluster)
        n203 = call "Enqueue Message.vi"("error in"=w397, "Data"=w394, "Message"="CalibParameters.Recalculate", "Queue"=w403) -> ("error out"=w400:errorcluster, "Queue dup."=w404:refnum<queue>)  [unwired: 6 in]
        n204 = call "Enqueue Message.vi"("error in"=w400, "Message"="Calib.Apply", "Queue"=w404) -> ("error out"=w399:errorcluster)  [unwired: 7 in, 1 out]
      }
      frame "CalibParameters.Recalculate" {
        w408 = refnum<vi> refnum  # Cluster
        n205 = Variant To Data(error in=w414, type=refnum<vi> refnum ("CtlRef"), Variant=w413) -> (data=w410:refnum<vi>, error out=w405:errorcluster)
        n206 = property class="DigNum (strict)"(reference=w410) -> ("Owner"=w409:refnum<vi>)  [unwired: 1 in, 2 out]
        n207 = To More Specific Class(target class=w408, reference=w409) -> (specific class reference=w407:refnum<vi>)  [unwired: 1 in, 1 out]
        n208 = property class="Clust"(reference=w407) -> ("Label.Text"=w406:string)  [unwired: 1 in, 2 out]
        n209 = case shown="\"Gain\"" w406 {
          tunnel: w410 -> [_ w432 w454 w485]
          tunnel: [w415 w428 w455 w499] -> w411
          tunnel: w405 -> [w415 _ _ w499]
          frame Default {
          }
          frame "Sensitivity" {
            n210 = control-ref of="Range"() -> (w431:refnum<vi>)
            n211 = property class="Clust (strict)"(reference=w431) -> ("Controls[]"=w430:refnum<vi>[])  [unwired: 1 in, 2 out]
            n212 = property class="DigNum (strict)"(reference=w432) -> ("Caption.Text"=w425:string, "Value"=w416:dbl)  [unwired: 1 in, 2 out]
            n213 = control-ref of="Voltage Limits"() -> (w427:refnum<vi>)
            n214 = property class="Clust (strict)"(reference=w427) -> ("Controls[]"=w426:refnum<vi>[])  [unwired: 1 in, 2 out]
            n215 = control-ref of="Gain"() -> (w422:refnum<vi>)
            n216 = property class="Clust (strict)"(reference=w422) -> ("Controls[]"=w421:refnum<vi>[])  [unwired: 1 in, 2 out]
            n217 = for {
              tunnel: w426 -> [w433] mode=indexing
              tunnel: w425 -> [w438]
              tunnel: [w436] -> w424
              stop <- w437 stop-if-true
              n218 = To More Specific Class(target class=refnum<vi> refnum ("X"), reference=w433) -> (specific class reference=w434:refnum<vi>)  [unwired: 1 in, 1 out]
              n219 = property class="DigNum (strict)"(reference=w434) -> (reference out=w436:refnum<vi>, "Caption.Text"=w439:string)  [unwired: 1 in, 1 out]
              n220 = Equal?(x=w439, y=w438) -> (x = y?=w437:bool)
            }
            n221 = for {
              tunnel: w430 -> [w444] mode=indexing
              tunnel: w425 -> [w448]
              tunnel: [w446] -> w429
              tunnel: w421 -> [w441] mode=indexing
              tunnel: [w440] -> w420
              stop <- w447 stop-if-true
              n222 = To More Specific Class(target class=refnum<vi> refnum ("X"), reference=w444) -> (specific class reference=w443:refnum<vi>)  [unwired: 1 in, 1 out]
              n223 = To More Specific Class(target class=refnum<vi> refnum ("X"), reference=w441) -> (specific class reference=w440:refnum<vi>)  [unwired: 1 in, 1 out]
              n224 = property class="DigNum (strict)"(reference=w443) -> (reference out=w446:refnum<vi>, "Caption.Text"=w449:string)  [unwired: 1 in, 1 out]
              n225 = Equal?(x=w449, y=w448) -> (x = y?=w447:bool)
            }
            n226 = property class="DigNum (strict)"(reference=w420) -> ("Value"=w419:dbl)  [unwired: 1 in, 2 out]
            n227 = property class="DigNum (strict)" props=["Value"](reference=w424) -> ()  [unwired: 1 in, 3 out]
            n228 = call "FGVfpgaAdress.vi"("Enum"=Enum."Read") -> ("voltageRange(+/-)Out"=w417:dbl)  [unwired: 5 in, 5 out]
            n229 = Compound Arithmetic op=MULTIPLY(w419, w416, w417) -> (w423:dbl)
            n230 = property class="DigNum (strict)"(reference=w429, "Value"=w423) -> (error out=w428:errorcluster)  [unwired: 1 in, 1 out]
          }
          frame "Range" {
            n231 = property class="DigNum (strict)"(reference=w454) -> ("Caption.Text"=w461:string, "Value"=w450:dbl)  [unwired: 1 in, 2 out]
            n232 = control-ref of="Sensitivity"() -> (w466:refnum<vi>)
            n233 = property class="Clust (strict)"(reference=w466) -> ("Controls[]"=w465:refnum<vi>[])  [unwired: 1 in, 2 out]
            n234 = control-ref of="Voltage Limits"() -> (w463:refnum<vi>)
            n235 = property class="Clust (strict)"(reference=w463) -> ("Controls[]"=w462:refnum<vi>[])  [unwired: 1 in, 2 out]
            n236 = control-ref of="Gain"() -> (w458:refnum<vi>)
            n237 = property class="Clust (strict)"(reference=w458) -> ("Controls[]"=w457:refnum<vi>[])  [unwired: 1 in, 2 out]
            n238 = for {
              tunnel: w462 -> [w467] mode=indexing
              tunnel: w461 -> [w472]
              tunnel: [w470] -> w460
              stop <- w471 stop-if-true
              n239 = To More Specific Class(target class=refnum<vi> refnum ("X"), reference=w467) -> (specific class reference=w468:refnum<vi>)  [unwired: 1 in, 1 out]
              n240 = property class="DigNum (strict)"(reference=w468) -> (reference out=w470:refnum<vi>, "Caption.Text"=w473:string)  [unwired: 1 in, 1 out]
              n241 = Equal?(x=w473, y=w472) -> (x = y?=w471:bool)
            }
            n242 = for {
              tunnel: w465 -> [w478] mode=indexing
              tunnel: w461 -> [w482]
              tunnel: [w480] -> w464
              tunnel: w457 -> [w475] mode=indexing
              tunnel: [w474] -> w456
              stop <- w481 stop-if-true
              n243 = To More Specific Class(target class=refnum<vi> refnum ("X"), reference=w478) -> (specific class reference=w477:refnum<vi>)  [unwired: 1 in, 1 out]
              n244 = To More Specific Class(target class=refnum<vi> refnum ("X"), reference=w475) -> (specific class reference=w474:refnum<vi>)  [unwired: 1 in, 1 out]
              n245 = property class="DigNum (strict)"(reference=w477) -> (reference out=w480:refnum<vi>, "Caption.Text"=w483:string)  [unwired: 1 in, 1 out]
              n246 = Equal?(x=w483, y=w482) -> (x = y?=w481:bool)
            }
            n247 = property class="DigNum (strict)"(reference=w460) -> ("Value"=w459:dbl)  [unwired: 1 in, 2 out]
            n248 = property class="DigNum (strict)"(reference=w456) -> ("Value"=w452:dbl)  [unwired: 1 in, 2 out]
            n249 = Compound Arithmetic op=MULTIPLY(w452, w459) -> (w451:dbl)
            n250 = Divide(x=w450, y=w451) -> (x/y=w453:dbl)
            n251 = property class="DigNum (strict)"(reference=w464, "Value"=w453) -> (error out=w455:errorcluster)  [unwired: 1 in, 1 out]
          }
          frame "Gain" {
            n252 = control-ref of="Range"() -> (w486:refnum<vi>)
            n253 = property class="Clust (strict)"(reference=w486) -> ("Controls[]"=w487:refnum<vi>[])  [unwired: 1 in, 2 out]
            n254 = property class="DigNum (strict)"(reference=w485) -> ("Caption.Text"=w491:string, "Value"=w484:dbl)  [unwired: 1 in, 2 out]
            n255 = control-ref of="Voltage Limits"() -> (w489:refnum<vi>)
            n256 = property class="Clust (strict)"(reference=w489) -> ("Controls[]"=w490:refnum<vi>[])  [unwired: 1 in, 2 out]
            n257 = control-ref of="Sensitivity"() -> (w495:refnum<vi>)
            n258 = property class="Clust (strict)"(reference=w495) -> ("Controls[]"=w496:refnum<vi>[])  [unwired: 1 in, 2 out]
            n259 = for {
              tunnel: w490 -> [w500] mode=indexing
              tunnel: w491 -> [w505]
              tunnel: [w503] -> w492
              stop <- w504 stop-if-true
              n260 = To More Specific Class(target class=refnum<vi> refnum ("X"), reference=w500) -> (specific class reference=w501:refnum<vi>)  [unwired: 1 in, 1 out]
              n261 = property class="DigNum (strict)"(reference=w501) -> (reference out=w503:refnum<vi>, "Caption.Text"=w506:string)  [unwired: 1 in, 1 out]
              n262 = Equal?(x=w506, y=w505) -> (x = y?=w504:bool)
            }
            n263 = for {
              tunnel: w487 -> [w511] mode=indexing
              tunnel: w491 -> [w515]
              tunnel: [w513] -> w488
              tunnel: w496 -> [w508] mode=indexing
              tunnel: [w507] -> w497
              stop <- w514 stop-if-true
              n264 = To More Specific Class(target class=refnum<vi> refnum ("X"), reference=w511) -> (specific class reference=w510:refnum<vi>)  [unwired: 1 in, 1 out]
              n265 = To More Specific Class(target class=refnum<vi> refnum ("X"), reference=w508) -> (specific class reference=w507:refnum<vi>)  [unwired: 1 in, 1 out]
              n266 = property class="DigNum (strict)"(reference=w510) -> (reference out=w513:refnum<vi>, "Caption.Text"=w516:string)  [unwired: 1 in, 1 out]
              n267 = Equal?(x=w516, y=w515) -> (x = y?=w514:bool)
            }
            n268 = property class="DigNum (strict)"(reference=w497) -> ("Value"=w498:dbl)  [unwired: 1 in, 2 out]
            n269 = property class="DigNum (strict)"(reference=w492) -> ("Value"=w494:dbl)  [unwired: 1 in, 2 out]
            n270 = Compound Arithmetic op=MULTIPLY(w498, w484, w494) -> (w493:dbl)
            n271 = property class="DigNum (strict)"(reference=w488, "Value"=w493) -> ()  [unwired: 1 in, 2 out]
          }
        }
      }
      frame "CalibParameters.SaveToFGV " {
      }
      frame "Analogs" {
        n272 = Variant To Data(error in=w525, type=refnum<vi> refnum ("CtlRef"), Variant=w526) -> (data=w523:refnum<vi>, error out=w522:errorcluster)
        n273 = property class="Clust (strict)"(reference=w523, error in=w522) -> (error out=w520:errorcluster, "Label.Text"=w527:string)  [unwired: 1 out]
        n274 = call "FGVfpgaAdress.vi"("Enum"=Enum."Read", "error in"=w520) -> ("error out"=w519:errorcluster, "FPGA VI Reference Out"=w518:T20)  [unwired: 4 in, 4 out]
        n275 = case shown="\"AI\"" w527 {
          tunnel: w518 -> [w532 w540]
          frame "AO", Default {
            n276 = property on="AO" class="Clust (strict)"() -> ("Value"=w528:T21)  [unwired: 2 in, 2 out]
            n277 = Cluster To Array(cluster=w528) -> (array=w531:bool[])
            n278 = Index Array(array=w531, index=2) -> (element=w530:bool)
            n279 = xnode "Read/Write Control"("FPGA VI Reference In"=w532, "aio.o.invertOutputs"=w531, "aio.o.invertHeight"=w530) -> ()  [unwired: 1 in, 2 out]
          }
          frame "AI" {
            n280 = property on="AI" class="Clust (strict)"() -> ("Value"=w533:T21)  [unwired: 2 in, 2 out]
            n281 = Cluster To Array(cluster=w533) -> (array=w539:bool[])
            n282 = Index Array(array=w539, index #1=0 ("index"), index #2=1 ("index")) -> (element #1=w536:bool, element #2=w535:bool)
            n283 = Build Array(w536, w535) -> (w534:bool[])
            n284 = xnode "Read/Write Control"("FPGA VI Reference In"=w540, "aio.o.invertInputs"=w539, "aio.o.invert2Inputs"=w534) -> ()  [unwired: 1 in, 2 out]
          }
        }
      }
      frame "Scanner.Configure" {
        # "Doesnt send the parameters to the FPGA"
        # "slow: 1 / False\nFast: 2 / True"
        n285 = Variant To Data(error in=w557, type=cluster{"CtlRef":refnum<vi>, "NewVal":variant} {"CtlRef"=refnum, "NewVal"=variant} ("output cluster"), Variant=w556) -> (data=w551:cluster{"CtlRef":refnum<vi>, "NewVal":variant}, error out=w548:errorcluster)
        n286 = Unbundle(w551) -> ("CtlRef"=w550:refnum<vi>, "NewVal"=w547:variant)
        n287 = property class="Ctl"(reference=w550) -> ("Label.Text"=w549:string)  [unwired: 1 in, 2 out]
        n288 = case shown="\"Speed config\"" w549 {
          tunnel: [w567 w582] -> w555
          tunnel: [w568 w579] -> w553
          tunnel: w548 -> [w573 w578]
          tunnel: w547 -> [w572 w577]
          frame "Time Constant (us)", Default {
            n289 = Variant To Data(error in=w573, type=TRUE, Variant=w572) -> (error out=w569:errorcluster)  [unwired: 1 out]
            n290 = call "FGVScannerConfig.vi"("Enum"=Enum."Read", "error in"=w569) -> ("error out"=w570:errorcluster, "scannerIdOut"=w567:i8)  [unwired: 7 in, 1 out]
            n291 = property on="Time Constant (us)" class="DigNum (strict)"(error in=w570) -> ("Value"=w568:u16)  [unwired: 1 in, 2 out]
          }
          frame "Speed config" {
            n292 = Variant To Data(error in=w578, type=TRUE, Variant=w577) -> (data=w575:bool)  [unwired: 1 out]
            n293 = Select(t=i8 2, s=w575, f=i8 1) -> (s? t:f=w582:i8)
            n294 = Select(t=u16 1000, s=w575, f=u16 40 ("t")) -> (s? t:f=w579:u16)
            n295 = property on="Time Constant (us)" class="DigNum (strict)"("Value"=w579) -> ()  [unwired: 2 in, 2 out]
          }
        }
        n296 = call "FGVScannerConfig.vi"("Enum"=Enum."Write", "scannerTimeConstantIn"=w553, "scannerIdIn"=w555) -> ("error out"=w543:errorcluster)  [unwired: 6 in, 2 out]
        n297 = call "IsVIRunning.vi"("error in (no error)"=w543, "name or relative path"="FrontPanel\\Excitation.vi") -> ("error out"=w546:errorcluster, "RunningVI?"=w545:bool)  [unwired: 8 in]
        n298 = case shown="True" w545 {
          tunnel: [w559 w566] -> w542
          tunnel: w546 -> [w559 w560]
          tunnel: w558 -> [_ w565]
          tunnel: "ScannerTimeConstant.Update" ("Message") -> [_ w564]
          frame False {
          }
          frame True {
            n299 = Obtain Queue(name (unnamed)="Excitation" ("QueueName"), element data type=T10 {"Message"="", "Données de message"=variant} ("Cluster Message"), error in (no error)=w560) -> (error out=w561:errorcluster)  [unwired: 2 in, 2 out]
            n300 = call "Enqueue Message.vi"("error in"=w561, "Message"=w564, "Queue"=w565) -> ("error out"=w566:errorcluster)  [unwired: 7 in, 1 out]
          }
        }
      }
      frame "HystCompensation.Update" {
        n301 = Variant To Data(error in=w590, type=TRUE, Variant=w589) -> (error out=w586:errorcluster)  [unwired: 1 out]
        n302 = call "FGVHysteresisCompensation.vi"("Enum"=Enum."Read", "error in"=w586) -> ("error out"=w585:errorcluster)  [unwired: 7 in, 2 out]
      }
      frame "Exit" {
        n303 = call "Fire User Event - Stop.vi"("Événement utilisateur - Arrêt"=w592) -> ("sortie d'erreur"=w591:errorcluster)  [unwired: 10 in]
        n304 = Release Queue(queue=w597, error in (no error)=w593) -> (error out=w595:errorcluster)  [unwired: 1 in, 2 out]
        n305 = Merge Errors(w591, w595) -> (w594:errorcluster)
      }
      frame Default {
        n306 = Format Into String(format string="The message\"%s\" received in the gestion loop is not valid" ("Texte de message d'erreur inconnu"), w601) -> (resulting string=w598:string)  [unwired: 2 in, 1 out]
        n307 = call <vilib>:"Error Cluster From Error Code.vi"("error message (\"\")"=w598, "error code (0)"=1 ("code d'erreur (0)")) -> ("error out"=w599:errorcluster)  [unwired: 7 in]
      }
    }
  }
  n308 = while {
    tunnel: w13 -> [w610]
    tunnel: [w606] -> w18
    shift-right: [w604] -> w19
    shift-left: w14 -> [w605]
    stop <- w608 stop-if-true
    n309 = event shown="[2] \"ActionsCalib.EditList.Apply\": Value Change" {
      selector: w605 -> [_ _ _ _ _ _ _ _ _ _ _]
      dyn-events: [_ _ _ _ _ _ _ _ _ _ _] -> w604
      timeout: _ -> [_ _ _ _ _ _ _ _ _ _ _]
      tunnel: [_ _ _ _ _ _ _ _ _ _ w667] -> w609
      tunnel: w610 -> [w620 w622 w625 w630 w636 w640 w645 w650 w656 w660 w666]
      tunnel: [_ _ _ w627 w631 _ w642 _ _ _ w665] -> w606
      tunnel: [w618 w622 w623 w628 w634 w638 w643 w648 w654 w659 w664] -> w607
      event "Actions": Edit Cell {
        n310 = event-data() -> ("String"=w617:string, "Row"=w616:i32)  [unwired: 1 in]
        n311 = property on="Menus" class="TabCtl (strict)"("Value"=w616) -> ()  [unwired: 2 in, 2 out]
        n312 = call "Enqueue Message.vi"("Data"=w617, "Message"="Actions.EditCell", "Queue"=w620) -> ("Queue dup."=w618:refnum<queue>)  [unwired: 7 in, 1 out]
      }
      event "Actions": Value Change {
        # "By selecting a new element in the list, open the page"
        n313 = event-data() -> ("NewVal"=w621:i32)  [unwired: 1 in]
        n314 = property on="Menus" class="TabCtl (strict)"("Value"=w621) -> ()  [unwired: 2 in, 2 out]
      }
      event "ActionsCalib.EditList.Apply": Value Change {
        n315 = event-data() -> ()  [unwired: 1 in, 1 out]
        n316 = call "Enqueue Message.vi"("Message"="ActionsCalib.EditList.Apply", "Queue"=w625) -> ("Queue dup."=w623:refnum<queue>)  [unwired: 8 in, 1 out]
      }
      event "ActionsCalib.Calibrations": Edit Cell {
        n317 = event-data() -> ("String"=w626:string)  [unwired: 1 in]
        n318 = call "Enqueue Message.vi"("Data"=w626, "Message"="CalibNames.Edit", "Queue"=w630) -> ("error out"=w627:errorcluster, "Queue dup."=w628:refnum<queue>)  [unwired: 7 in]
      }
      event "ActionsCalib.EditList.Delete", "ActionsCalib.EditList.Up", "ActionsCalib.EditList.Down", "ActionsCalib.EditList.Copy", "ActionsCalib.EditList.Add": Mouse Down {
        n319 = event-data() -> ("CtlRef"=w633:refnum<vi>)  [unwired: 1 in]
        n320 = property class="Bool (strict)"(reference=w633) -> ("Label.Text"=w632:string)  [unwired: 1 in, 2 out]
        n321 = call "Enqueue Message.vi"("Data"=w632, "Message"="CalibName.EditList", "Queue"=w636) -> ("error out"=w631:errorcluster, "Queue dup."=w634:refnum<queue>)  [unwired: 7 in]
      }
      event "ActionsCalib.Calibrations": Value Change {
        n322 = event-data() -> ("NewVal"=w637:i32)  [unwired: 1 in]
        n323 = call "Enqueue Message.vi"("Data"=w637, "Message"="Calibration.ChangeDisplay", "Queue"=w640) -> ("Queue dup."=w638:refnum<queue>)  [unwired: 7 in, 1 out]
      }
      event "ActionsCalib.Calib parameters.Sensitivity.Sens X", "ActionsCalib.Calib parameters.Sensitivity.Sens Y", "ActionsCalib.Calib parameters.Sensitivity.Sens Z", "ActionsCalib.Calib parameters.Range.Range X", "ActionsCalib.Calib parameters.Range.Range Y", "ActionsCalib.Calib parameters.Range.Range Z", "ActionsCalib.Calib parameters.Gain.HV gain X", "ActionsCalib.Calib parameters.Gain.HV gain Y", "ActionsCalib.Calib parameters.Gain.HV gain Z": Value Change {
        n324 = event-data() -> ("CtlRef"=w641:refnum<vi>)  [unwired: 1 in]
        n325 = call "Enqueue Message.vi"("Data"=w641, "Message"="CalibParameters.Update", "Queue"=w645) -> ("error out"=w642:errorcluster, "Queue dup."=w643:refnum<queue>)  [unwired: 7 in]
      }
      event "Analogs.AI", "Analogs.AO": Value Change {
        n326 = event-data() -> ("CtlRef"=w647:refnum<vi>)  [unwired: 1 in, 2 out]
        n327 = To Variant(anything=w647) -> (Variant=w646:variant)
        n328 = call "Enqueue Message.vi"("Data"=w646, "Message"="Analogs", "Queue"=w650) -> ("Queue dup."=w648:refnum<queue>)  [unwired: 7 in, 1 out]
      }
      event "ScannerConfig.Speed config", "ScannerConfig.Time Constant (us)": Value Change {
        n329 = event-data() -> ("CtlRef"=w653:refnum<vi>, "NewVal"=w652:variant)  [unwired: 1 in]
        n330 = Bundle("CtlRef"=w653, "NewVal"=w652) -> (w651:cluster{"CtlRef":refnum<vi>, "NewVal":variant})  [unwired: 1 in]
        n331 = call "Enqueue Message.vi"("Data"=w651, "Message"="Scanner.Configure", "Queue"=w656) -> ("Queue dup."=w654:refnum<queue>)  [unwired: 7 in, 1 out]
      }
      event "Hyst Compens.Hysteresis Comp": Value Change {
        n332 = event-data() -> ("NewVal"=w657:bool)  [unwired: 1 in]
        n333 = call "Enqueue Message.vi"("Data"=w657, "Message"="HystCompensation.Update", "Queue"=w660) -> ("Queue dup."=w659:refnum<queue>)  [unwired: 7 in, 1 out]
      }
      event Panel Close? {
        w667 = TRUE ("Rejeter ?")
        n334 = event-data() -> ()  [unwired: 1 in, 1 out]
        n335 = Flush Queue(queue=w666) -> (queue out=w669:refnum<queue>)  [unwired: 1 in, 2 out]
        n336 = disable-structure shown="Disabled" {
          disable-tunnel: [w676 _] -> w661
          frame Disabled {
            n337 = call "FGVSessionPath.vi"("Enum"=Enum."Read") -> ("sessionPathOut"=w679:path)  [unwired: 9 in, 1 out]
            n338 = Build Path(base path=w679, name or relative path="SettingsCalib.txt") -> (appended path=w676:path)
          }
          frame Enabled {
          }
        }
        n339 = disable-structure shown="Disabled" {
          disable-tunnel: w669 -> [w674 w675]
          disable-tunnel: [w673 w675] -> w668
          disable-tunnel: [w672 _] -> w662
          disable-tunnel: w661 -> [w671 _]
          frame Disabled {
            (unwired) "Configuration.Write" ("Message")
            n340 = call "Enqueue Message.vi"("Data"=w671, "Message"="", "Queue"=w674) -> ("error out"=w672:errorcluster, "Queue dup."=w673:refnum<queue>)  [unwired: 7 in]
          }
          frame Enabled {
          }
        }
        n341 = event-data ("Event Filter Node")("Discard?"=w667) -> ()  [unwired: 1 in, 1 out]
        n342 = call "Enqueue Message.vi"("error in"=w662, "Message"="Exit", "Queue"=w668) -> ("error out"=w665:errorcluster, "Queue dup."=w664:refnum<queue>)  [unwired: 7 in]
      }
    }
    n343 = case shown="Error" w606 {
      tunnel: [w611 TRUE ("Rejeter ?")] -> w608
      tunnel: w609 -> [w611 _]
      tunnel: w607 -> [_ w614]
      frame No Error {
      }
      frame Error {
        n344 = call "Enqueue Message.vi"("Prioritary message"=TRUE ("Message prioritaire ? (F)"), "Message"="Exit", "Queue"=w614) -> ()  [unwired: 7 in, 2 out]
      }
    }
    n345 = Wait (ms)(milliseconds to wait=u32 200) -> ()  [unwired: 1 out]
  }
  n346 = Unregister For Events(event registration refnum=w19, error in=w18) -> (error out=w20:errorcluster)
  n347 = Merge Errors(w20, w12) -> (w16:errorcluster)
  n348 = call "Destroy User Event - Stop.vi"("entrée d'erreur (pas d'erreur)"=w16, "Événement utilisateur - Arrêt"=w17) -> ("sortie d'erreur"=w15:errorcluster)  [unwired: 9 in]
  n349 = call <vilib>:"Simple Error Handler.vi"("error in (no error)"=w15) -> ("error out"=w2:errorcluster)  [unwired: 4 in, 4 out]
  n350 = call "FGVFileServer.vi"("Enum"=EnumFGVHDT."Pop", "error in"=w2, "New VI"=w21) -> ()  [unwired: 7 in, 2 out]
